vi "stage_xyz_gui.vi"() -> ()   [LabVIEW 2014]
uses:
  <vilib>/Utility/miscctls.llb/LVPointDoubleTypeDef.ctl
  D:/Microscope/Software/Tools/Stage_xyz/Dll/Newport.CONEXCC.CommandInterface.dll
  Tools/Stage_xyz/Dll/Newport.CONEXCC.CommandInterface.dll
panel:
  in  "y_max":dbl=20.0 caption="Y:" min=0.0 max=25.0 format="%#.3f"
  in  "x_max":dbl=20.0 caption="X:" min=0.0 max=25.0 format="%#.3f"
  in  "y_min":dbl caption="Y:" min=0.0 max=25.0 format="%#.3f"
  in  "x_min":dbl caption="X:" min=0.0 max=25.0 format="%#.3f"
  in  "speed_z":dbl=0.4 caption="Z:" min=0.0 max=25.0 format="%#.3f"
  in  "speed_xy":dbl=0.4 caption="X, Y:" min=0.0 max=25.0 format="%#.3f"
  out "status_z":bool
  out "status_y":bool
  out "status_x":bool
  in  "com_z":string(combo)="COM6" caption="Z:"
  in  "com_y":string(combo)="COM5" caption="Y:"
  in  "com_x":string(combo)="COM7" caption="X:"
  in  "increment":dbl=0.01 caption="Increment [mm]" min=0.0 max=25.0 step=0.001 format="%.3f"
  out "current_speed_z":dbl=0.4 caption="Z:" min=0.0 max=25.0 format="%#.3f"
  out "current_speed_x":dbl=0.4 caption="X:" min=0.0 max=25.0 format="%#.3f"
  out "position_z":dbl format="%#.3f"
  out "position_y":dbl format="%#.3f"
  out "position_x":dbl format="%#.3f"
  out "state_x":u32 caption="X:"
  out "state_y":u32 caption="Y:"
  out "state_z":u32 caption="Z:"
  out "current_speed_y":dbl=0.4 caption="Y:" min=0.0 max=25.0 format="%#.3f"
  in  "stop_move":bool
  out "xy_position":cluster{"X":dbl, "Y":dbl}[](graph)
  in  "x_val":dbl caption="X:" min=0.0 max=20.0 format="%.3g"
  in  "y_val":dbl caption="Y:" min=0.0 max=20.0 format="%.3g"
  in  "stop":bool
  # "Min."
  # "Max."
  # "[mm]"
  # "Speed [mm/s]"
  # "State:"
  # "Position:"
  # "Speed:"
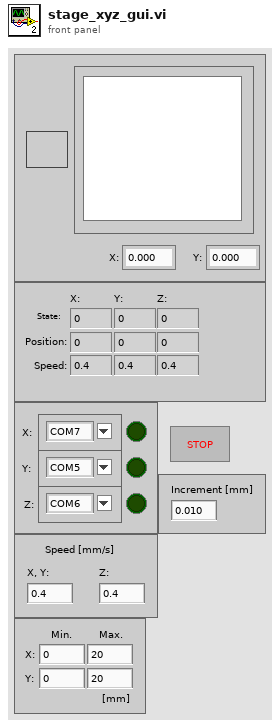
[diagram p1: front panel]
types:
  T1 = typedef "LVPointDoubleTypeDef.ctl" = cluster{"X":dbl, "Y":dbl}
  T2 = cluster{"com_x":string, "com_y":string, "com_z":string}
  T3 = cluster{"conn_x":refnum<k24>, "conn_y":refnum<k24>, "conn_z":refnum<k24>}
  T4 = cluster{"conn_x_out":refnum<k24>, "conn_y_out":refnum<k24>, "conn_z_out":refnum<k24>}
  T5 = enum16{"Standby", "Goto", "Stop", "Status", "Goto_z"}
  T6 = typedef "eventvkey.ctl" = enum16{"ASCII", "Enter", "Return", "Shift", "Ctrl", "Alt", "Cmd", "Opt", "Caps", "NumLock", "Clear", "Break", "Up", "Down", "Left", "Right", "Insert", "Delete", "Home", "End", "PageUp", "PageDown", "Escape", "Help", "Pause", "ScrollLock", "F1", "F2", "F3", "F4", "F5", "F6", "F7", "F8", "F9", "F10", "F11", "F12", "F13", "F14", "F15", "F16", "F17", "F18", "F19", "F20", "F21", "F22", "F23", "F24", "Play", "VolumeUp", "VolumeDown", "Mute", "Two Byte Char"}
  T7 = cluster{"CurrentPosition":dbl, "CurrentPosition":dbl, "CurrentPosition":dbl}
  T8 = cluster{"controllerState":u32, "controllerState":u32, "controllerState":u32}
  T9 = cluster{"Velocity":dbl, "Velocity":dbl, "Velocity":dbl}
  T10 = cluster{"CurrentPosition":dbl, "CurrentPosition":dbl}
  T11 = cluster{"CurrentPosition":dbl, "CurrentPosition":dbl}[]
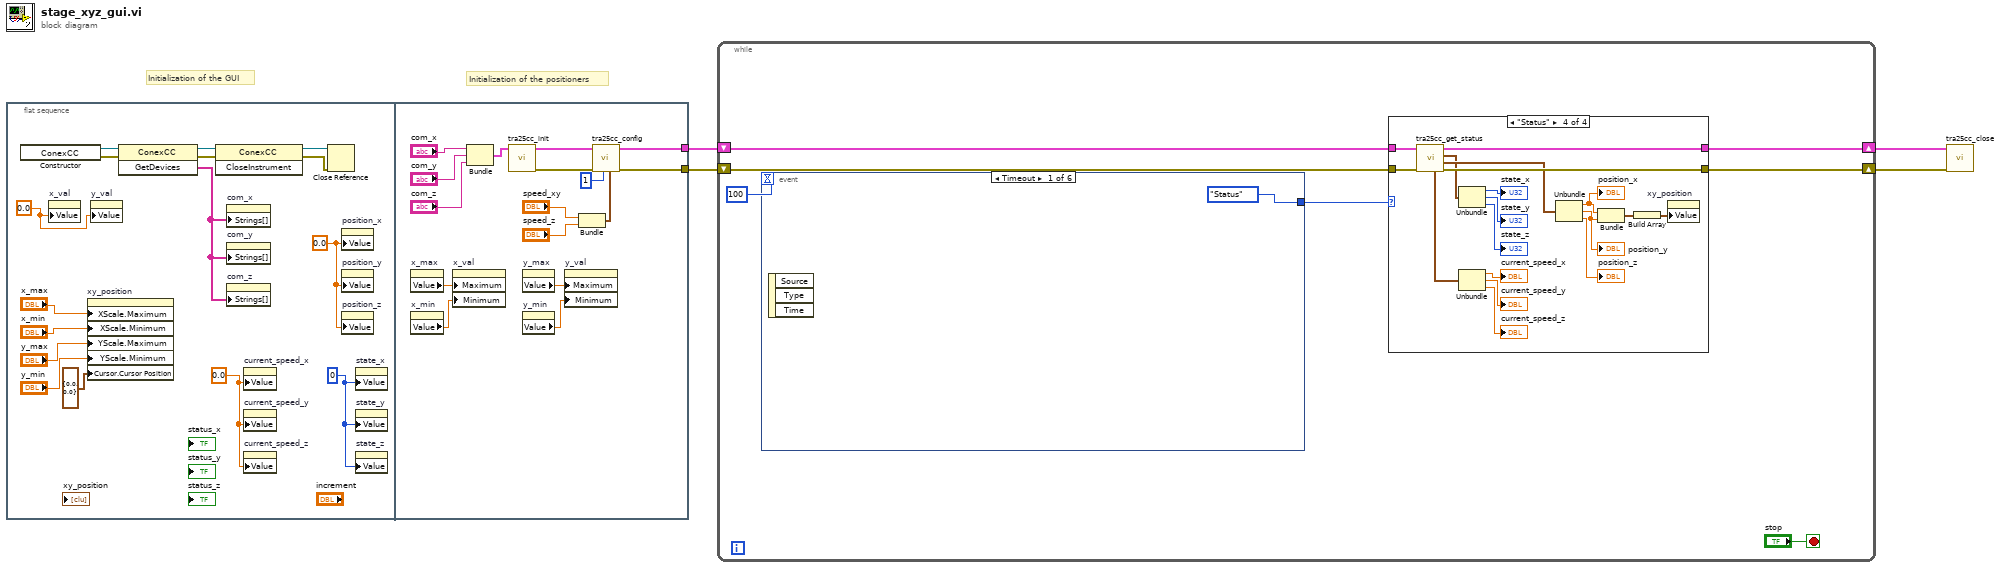
[diagram p0: block diagram]
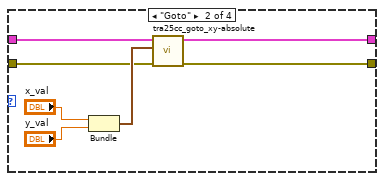
[diagram p3: hidden frame]
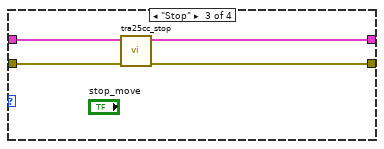
[diagram p4: hidden frame]
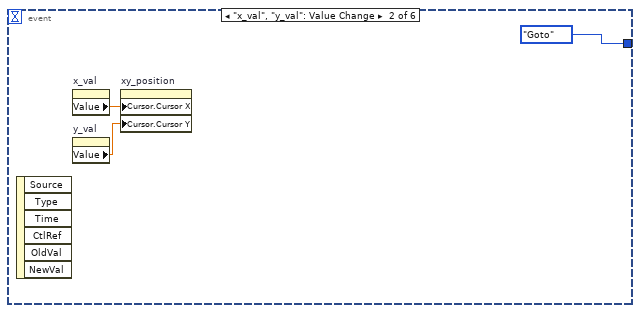
[diagram p5: hidden frame]
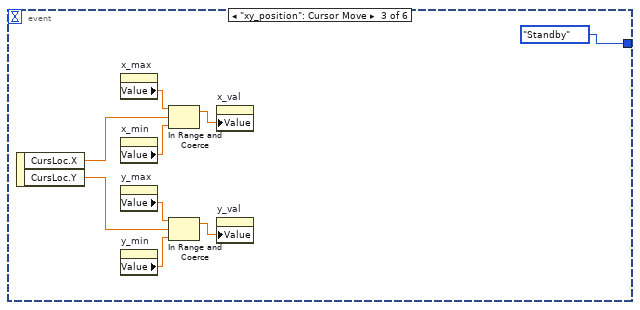
[diagram p6: hidden frame]
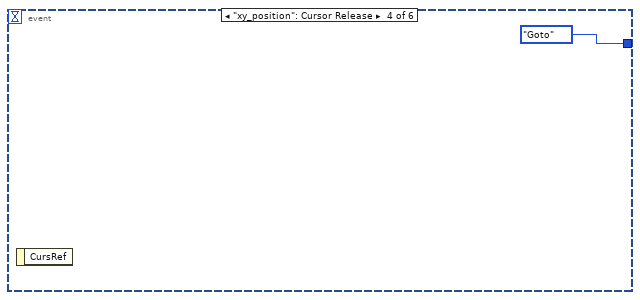
[diagram p7: hidden frame]
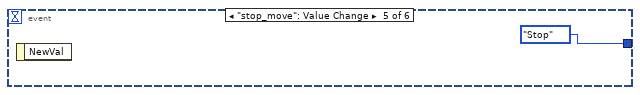
[diagram p8: hidden frame]
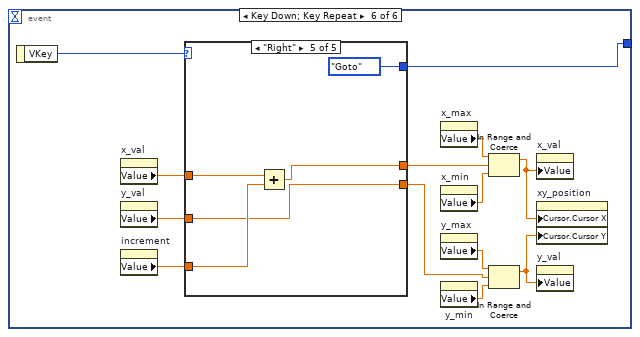
[diagram p9: hidden frame]
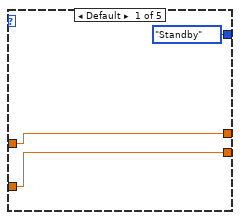
[diagram p10: hidden frame]
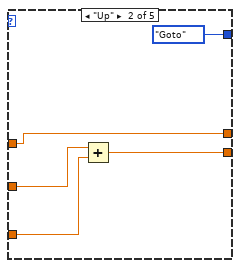
[diagram p11: hidden frame]
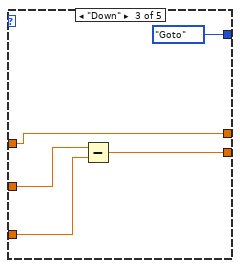
[diagram p12: hidden frame]
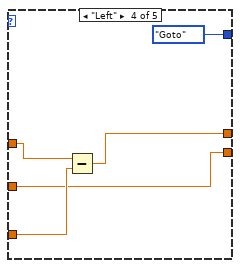
[diagram p13: hidden frame]
diagram:
  # "Initialization of the positioners"
  # "Initialization of the GUI"
  n1 = flat-sequence {
    tunnel: [w35] -> w4
    tunnel: [w34] -> w1
    frame #0 {
      w5 = 0.0 ("position_x")
      w6 = u32 0 ("state_x")
      w7 = 0.0 ("current_speed_x")
      w13 = 0.0 ("x_val")
      n2 = constructor class="ConexCC"() -> (reference out=w20:refnum<k24>, error out=w18:errorcluster)  [unwired: 3 in, 1 out]
      n3 = property on="x_val" class="DigNum (strict)"("Value"=w13) -> ()  [unwired: 2 in, 2 out]
      n4 = property on="xy_position" class="XYGraph (strict)"("XScale.Maximum"="x_max", "XScale.Minimum"="x_min", "YScale.Maximum"="y_max", "YScale.Minimum"="y_min", "Cursor.Cursor Position"=T1 {"X"=0.0, "Y"=0.0}) -> ()  [unwired: 2 in, 2 out]
      n5 = property on="y_val" class="DigNum (strict)"("Value"=w13) -> ()  [unwired: 2 in, 2 out]
      n6 = invoke class="ConexCC" method="GetDevices"(reference=w20, error in=w18) -> (reference out=w15:refnum<k24>, error out=w14:errorcluster, "GetDevices"=w19:string[])  [unwired: 1 in]
      n7 = invoke class="ConexCC" method="CloseInstrument"(reference=w15, error in=w14) -> (reference out=w17:refnum<k24>, error out=w16:errorcluster)  [unwired: 1 in, 1 out]
      n8 = property on="com_x" class="CmbBox"("Strings[]"=w19) -> ()  [unwired: 2 in, 2 out]
      n9 = property on="com_y" class="CmbBox"("Strings[]"=w19) -> ()  [unwired: 2 in, 2 out]
      n10 = property on="com_z" class="CmbBox"("Strings[]"=w19) -> ()  [unwired: 2 in, 2 out]
      n11 = property on="current_speed_x" class="DigNum (strict)"("Value"=w7) -> ()  [unwired: 2 in, 2 out]
      n12 = property on="current_speed_y" class="DigNum (strict)"("Value"=w7) -> ()  [unwired: 2 in, 2 out]
      n13 = property on="current_speed_z" class="DigNum (strict)"("Value"=w7) -> ()  [unwired: 2 in, 2 out]
      n14 = Close Reference(reference=w17, error in (no error)=w16) -> ()  [unwired: 1 out]
      n15 = property on="position_x" class="DigNum (strict)"("Value"=w5) -> ()  [unwired: 2 in, 2 out]
      n16 = property on="position_y" class="DigNum (strict)"("Value"=w5) -> ()  [unwired: 2 in, 2 out]
      n17 = property on="position_z" class="DigNum (strict)"("Value"=w5) -> ()  [unwired: 2 in, 2 out]
      n18 = property on="state_x" class="DigNum (strict)"("Value"=w6) -> ()  [unwired: 2 in, 2 out]
      n19 = property on="state_y" class="DigNum (strict)"("Value"=w6) -> ()  [unwired: 2 in, 2 out]
      n20 = property on="state_z" class="DigNum (strict)"("Value"=w6) -> ()  [unwired: 2 in, 2 out]
    }
    frame #1 {
      n21 = property on="x_max" class="DigNum (strict)"() -> ("Value"=w24:dbl)  [unwired: 2 in, 2 out]
      n22 = property on="x_min" class="DigNum (strict)"() -> ("Value"=w23:dbl)  [unwired: 2 in, 2 out]
      n23 = property on="x_val" class="DigNum (strict)"("Maximum"=w24, "Minimum"=w23) -> ()  [unwired: 2 in, 2 out]
      n24 = Bundle("com_x"="com_x", "com_y"="com_y", "com_z"="com_z") -> (w30:T2)  [unwired: 1 in]
      n25 = call "tra25cc_init.vi"("com_xyz"=w30) -> ("error IO"=w36:errorcluster, "conn_xyz"=w29:T3)  [unwired: 9 in]
      n26 = property on="y_max" class="DigNum (strict)"() -> ("Value"=w22:dbl)  [unwired: 2 in, 2 out]
      n27 = property on="y_min" class="DigNum (strict)"() -> ("Value"=w21:dbl)  [unwired: 2 in, 2 out]
      n28 = property on="y_val" class="DigNum (strict)"("Maximum"=w22, "Minimum"=w21) -> ()  [unwired: 2 in, 2 out]
      n29 = Bundle("speed_xy"="speed_xy", "speed_z"="speed_z") -> (w25:cluster{"speed_xy":dbl, "speed_z":dbl})  [unwired: 1 in]
      n30 = call "tra25cc_config.vi"("speed_xyz"=w25, "tracking mode"=1, "error in (no error)"=w36, "conn_xyz_in"=w29) -> ("error out"=w34:errorcluster, "conn_xyz_out"=w35:T4)  [unwired: 6 in]
    }
  }
  n31 = while {
    shift-right: [w39] -> w3
    shift-left: w4 -> [w40]
    shift-right: [w38] -> w2
    shift-left: w1 -> [w41]
    stop <- "stop" stop-if-true
    n32 = event shown="[0] Timeout" {
      selector: _ -> [_ _ _ _ _ _]
      dyn-events: _ -> [_ _ _ _ _ _]
      timeout: 100 -> [_ _ _ _ _ _]
      tunnel: [T5."Status" T5."Goto" T5."Standby" T5."Goto" T5."Stop" w90] -> w42
      event Timeout {
        n33 = event-data() -> ()  [unwired: 1 in, 3 out]
      }
      event "x_val", "y_val": Value Change {
        n34 = event-data() -> ()  [unwired: 1 in, 6 out]
        n35 = property on="x_val" class="DigNum (strict)"() -> ("Value"=w78:dbl)  [unwired: 2 in, 2 out]
        n36 = property on="y_val" class="DigNum (strict)"() -> ("Value"=w77:dbl)  [unwired: 2 in, 2 out]
        n37 = property on="xy_position" class="XYGraph (strict)"("Cursor.Cursor X"=w78, "Cursor.Cursor Y"=w77) -> ()  [unwired: 2 in, 2 out]
      }
      event "xy_position": Cursor Move {
        n38 = event-data() -> ("CursLoc.X"=w81:dbl, "CursLoc.Y"=w80:dbl)  [unwired: 1 in]
        n39 = property on="x_max" class="DigNum (strict)"() -> ("Value"=w83:dbl)  [unwired: 2 in, 2 out]
        n40 = property on="x_min" class="DigNum (strict)"() -> ("Value"=w84:dbl)  [unwired: 2 in, 2 out]
        n41 = property on="y_max" class="DigNum (strict)"() -> ("Value"=w82:dbl)  [unwired: 2 in, 2 out]
        n42 = property on="y_min" class="DigNum (strict)"() -> ("Value"=w85:dbl)  [unwired: 2 in, 2 out]
        n43 = In Range and Coerce(upper limit=w83, x=w81, lower limit=w84) -> (coerced(x)=w87:dbl)  [unwired: 1 out]
        n44 = In Range and Coerce(upper limit=w82, x=w80, lower limit=w85) -> (coerced(x)=w86:dbl)  [unwired: 1 out]
        n45 = property on="x_val" class="DigNum (strict)"("Value"=w87) -> ()  [unwired: 2 in, 2 out]
        n46 = property on="y_val" class="DigNum (strict)"("Value"=w86) -> ()  [unwired: 2 in, 2 out]
      }
      event "xy_position": Cursor Release {
        n47 = event-data() -> ()  [unwired: 1 in, 1 out]
      }
      event "stop_move": Value Change {
        n48 = event-data() -> ()  [unwired: 1 in, 1 out]
      }
      event Key Down; Key Repeat {
        n49 = event-data() -> ("VKey"=w102:T6)  [unwired: 1 in]
        n50 = property on="x_val" class="DigNum (strict)"() -> ("Value"=w95:dbl)  [unwired: 2 in, 2 out]
        n51 = property on="y_val" class="DigNum (strict)"() -> ("Value"=w94:dbl)  [unwired: 2 in, 2 out]
        n52 = property on="increment" class="DigNum (strict)"() -> ("Value"=w93:dbl)  [unwired: 2 in, 2 out]
        n53 = case shown="\"Right\"" w102 {
          tunnel: [w105 w107 w112 w118 w123] -> w97
          tunnel: [w104 w108 w114 w117 w122] -> w96
          tunnel: w95 -> [w105 w107 w112 w119 w125]
          tunnel: w94 -> [w104 w109 w113 w117 w122]
          tunnel: w93 -> [_ w110 w115 w120 w124]
          tunnel: [T5."Standby" T5."Goto" T5."Goto" T5."Goto" T5."Goto"] -> w90
          frame Default {
          }
          frame "Up" {
            n54 = Add(x=w109, y=w110) -> (x+y=w108:dbl)
          }
          frame "Down" {
            n55 = Subtract(x=w113, y=w115) -> (x-y=w114:dbl)
          }
          frame "Left" {
            n56 = Subtract(x=w119, y=w120) -> (x-y=w118:dbl)
          }
          frame "Right" {
            n57 = Add(x=w125, y=w124) -> (x+y=w123:dbl)
          }
        }
        n58 = property on="x_max" class="DigNum (strict)"() -> ("Value"=w101:dbl)  [unwired: 2 in, 2 out]
        n59 = property on="x_min" class="DigNum (strict)"() -> ("Value"=w100:dbl)  [unwired: 2 in, 2 out]
        n60 = property on="y_max" class="DigNum (strict)"() -> ("Value"=w99:dbl)  [unwired: 2 in, 2 out]
        n61 = property on="y_min" class="DigNum (strict)"() -> ("Value"=w98:dbl)  [unwired: 2 in, 2 out]
        n62 = In Range and Coerce(upper limit=w101, x=w97, lower limit=w100) -> (coerced(x)=w92:dbl)  [unwired: 1 out]
        n63 = In Range and Coerce(upper limit=w99, x=w96, lower limit=w98) -> (coerced(x)=w91:dbl)  [unwired: 1 out]
        n64 = property on="x_val" class="DigNum (strict)"("Value"=w92) -> ()  [unwired: 2 in, 2 out]
        n65 = property on="xy_position" class="XYGraph (strict)"("Cursor.Cursor X"=w92, "Cursor.Cursor Y"=w91) -> ()  [unwired: 2 in, 2 out]
        n66 = property on="y_val" class="DigNum (strict)"("Value"=w91) -> ()  [unwired: 2 in, 2 out]
      }
    }
    n67 = case shown="\"Status\"" w42 {
      tunnel: [w45 w49 w55 w72] -> w39
      tunnel: [w44 w46 w53 w71] -> w38
      tunnel: w40 -> [w45 w50 w56 w74]
      tunnel: w41 -> [w44 w47 w54 w73]
      frame "Standby", Default {
      }
      frame "Goto" {
        n68 = Bundle("x_val"="x_val", "y_val"="y_val") -> (w48:cluster{"x_val":dbl, "y_val":dbl})  [unwired: 1 in]
        n69 = call "tra25cc_goto_xy-absolute.vi"("error in (no error)"=w47, "xy_val"=w48, "conn_xyz_in"=w50) -> ("error out"=w46:errorcluster, "conn_xyz_out"=w49:T4)  [unwired: 7 in]
      }
      frame "Stop" {
        n70 = call "tra25cc_stop.vi"("error in (no error)"=w54, "conn_xyz_in"=w56) -> ("error out"=w53:errorcluster, "conn_xyz_out"=w55:T4)  [unwired: 8 in]
      }
      frame "Status" {
        n71 = call "tra25cc_get_status.vi"("error in (no error)"=w73, "conn_xyz_in"=w74) -> ("error out"=w71:errorcluster, "position_xyz"=w68:T7, "state_xyz"=w62:T8, "conn_xyz_out"=w72:T4, "current_speed_xyz"=w70:T9)  [unwired: 5 in]
        n72 = Unbundle(w62) -> ("controllerState"=→"state_x":u32, "controllerState"=→"state_y":u32, "controllerState"=→"state_z":u32)
        n73 = Unbundle(w70) -> ("Velocity"=→"current_speed_x":dbl, "Velocity"=→"current_speed_y":dbl, "Velocity"=→"current_speed_z":dbl)
        n74 = Unbundle(w68) -> ("CurrentPosition"=w66:dbl, "CurrentPosition"=w65:dbl, "CurrentPosition"=→"position_z":dbl)
        "position_x" <- w66
        "position_y" <- w65
        n75 = Bundle("CurrentPosition"=w66, "CurrentPosition"=w65) -> (w67:T10)  [unwired: 1 in]
        n76 = Build Array(w67) -> (w64:T11)
        n77 = property on="xy_position" class="XYGraph (strict)"("Value"=w64) -> ()  [unwired: 2 in, 2 out]
      }
    }
  }
  n78 = call "tra25cc_close.vi"("error in (no error)"=w2, "conn_xyz_in"=w3) -> ()  [unwired: 9 in, 1 out]
